vi "Configure.vi"(8 "error in (no error)":errorcluster, 10 "Msg in":T1, 11 "FakePressureController in":refnum<class "TapeMonitor.lvclass">) -> (0 "error out":errorcluster, 1 "new command":string, 2 "Msg out":T1, 3 "FakePressureController out":refnum<class "TapeMonitor.lvclass">)   [LabVIEW 2013, in "TapeMonitor.lvclass"]
uses:
  TapeMonitor.lvclass
  DriverMsg.ctl
  TapeMonitor.lvclass/TapeMonitor.ctl
  OnOffTypeDef.ctl
  source/Device Driver/BaseDriver/BaseDriver.lvclass
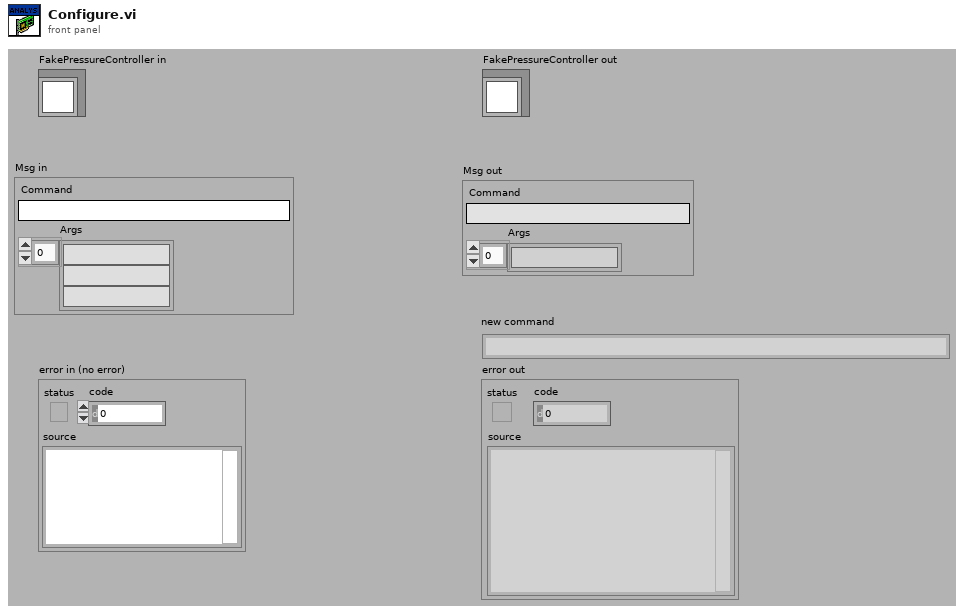
[diagram p1: front panel]
types:
  T1 = typedef "DriverMsg.ctl" = cluster{"Command":string, "Args":string[]}
  T2 = typedef "OnOffTypeDef.ctl" = enum16{"off", "on"}
  T3 = typedef "TapeMonitor.lvclass/settings_TypDef.ctl" = cluster{"timeout":T4, "FitnessLimit":T4, "LocalSavingPath":path, "Save":T2, "threshold_low":T4, "threshold_high":T4, "area_min":T4, "area_max":T4}
  T4 = typedef "BaseDriver.lvclass/numericVariable_TypeDef.ctl" = cluster{"Value":dbl, "Min":dbl, "Max":dbl, "StepSize":dbl, "Tolerance":dbl, "ValueActual":dbl}
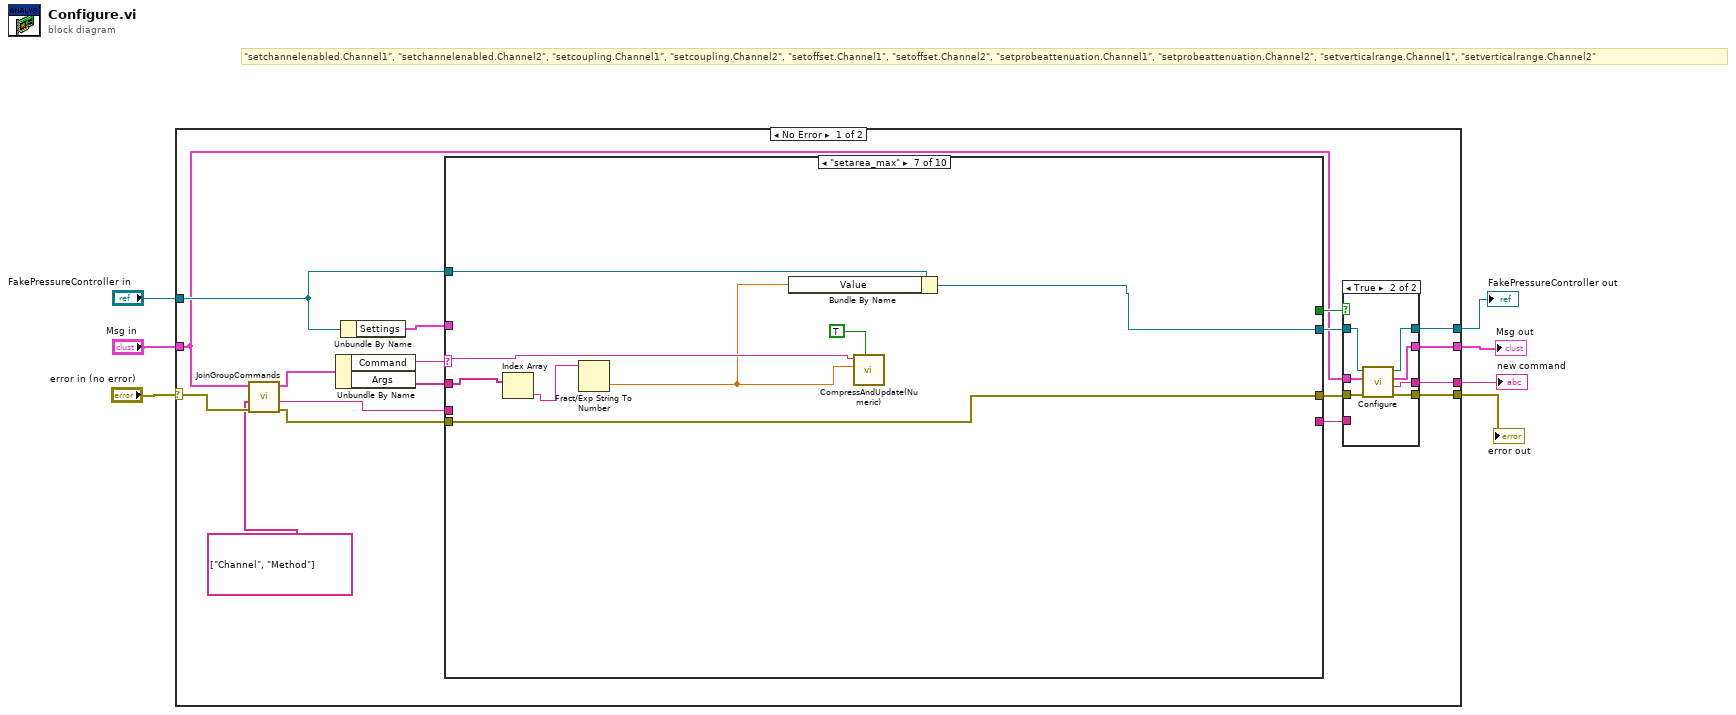
[diagram p0: block diagram]
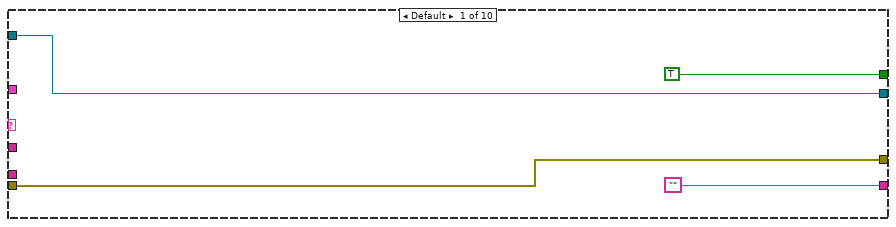
[diagram p3: hidden frame]
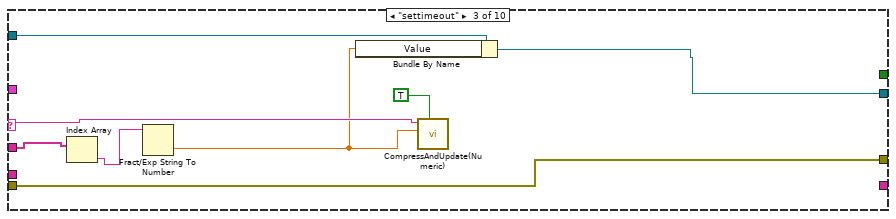
[diagram p5: hidden frame]
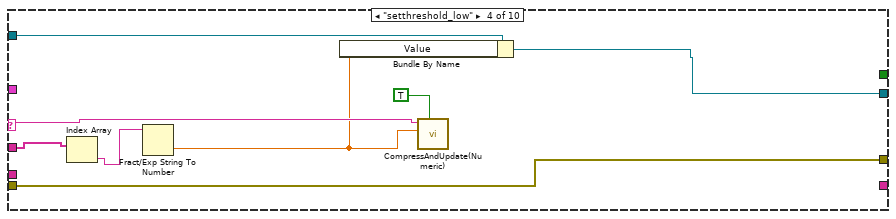
[diagram p6: hidden frame]
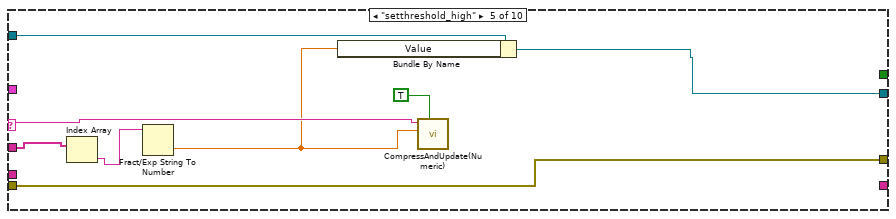
[diagram p7: hidden frame]
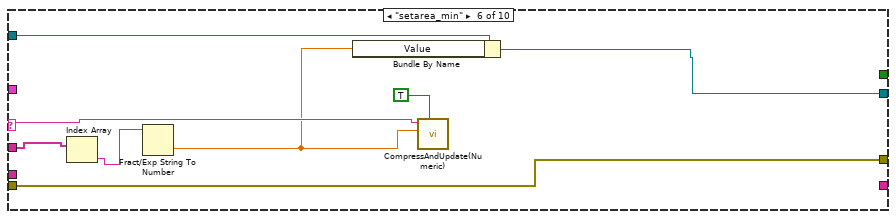
[diagram p8: hidden frame]
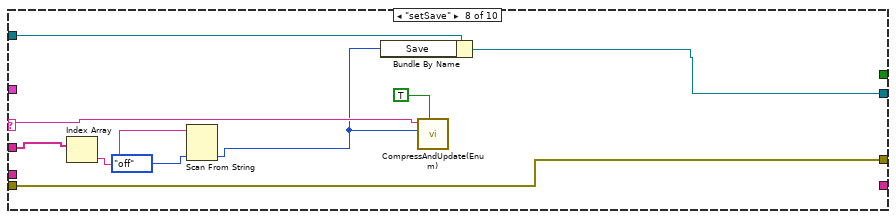
[diagram p9: hidden frame]
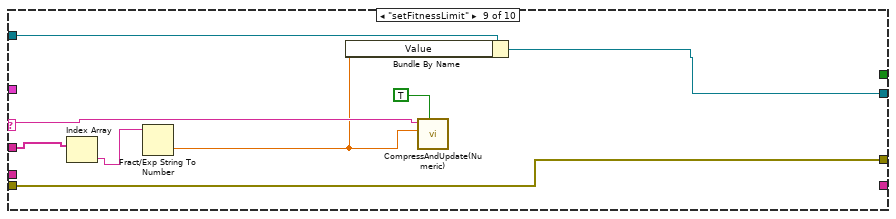
[diagram p10: hidden frame]
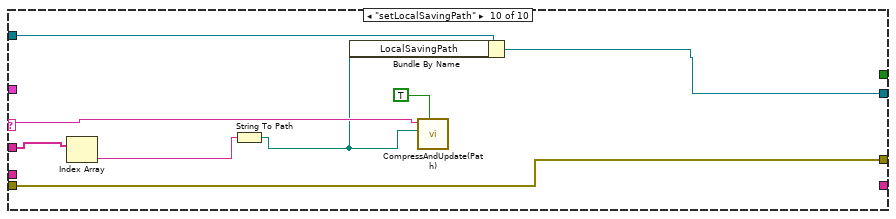
[diagram p11: hidden frame]
diagram:
  # "\"setchannelenabled.Channel1\", \"setchannelenabled.Channel2\", \"setcoupling.Channel1\", \"setcoupling.Channel2\", \"setoffset.Channel1\", \"setoffset.Channel2\", \"setprobeattenuation.Channel1\", \"setprobeattenuation.Channel2\", \"setverticalrange.Channel1\", \"setverticalrange.Channel2\""
  n1 = case shown="No Error" "error in (no error)" {
    selector: "error in (no error)" -> [w13 w110]
    tunnel: "FakePressureController in" -> [w16 w108]
    tunnel: [w24 w108] -> w4
    tunnel: [w22 w110] -> w1
    tunnel: "Msg in" -> [w10 w109]
    tunnel: [w20 w109] -> w3
    tunnel: [w18 _] -> w2
    frame No Error {
      n2 = call "JoinGroupCommands.vi"("error in (no error)"=w13, "Seperator"=string[] ["Channel", "Method"], "Msg in"=w10) -> ("error out"=w12:errorcluster, "Seperator out"=w9:string, "Msg out"=w11:T1)  [unwired: 6 in]
      n3 = Unbundle By Name(w11) -> ("Command"=w17:string, "Args"=w14:string[])
      n4 = Unbundle By Name(w16) -> ("Settings"=w15:T3)
      n5 = case shown="\"setarea_max\"" w17 {
        selector: w17 -> [_ _ w44 w52 w60 w68 w76 w86 w93 w102]
        tunnel: w12 -> [w39 w41 w50 w58 w66 w74 w82 w91 w99 w107]
        tunnel: w14 -> [_ _ w49 w57 w65 w73 w81 w90 w98 w106]
        tunnel: w16 -> [w40 w42 w47 w55 w63 w71 w79 w89 w96 w105]
        tunnel: [w40 w42 w46 w54 w62 w70 w78 w88 w95 w104] -> w25
        tunnel: ["" ("Complete") _ _ _ _ _ _ _ _ _] -> w19
        tunnel: [w39 w41 w50 w58 w66 w74 w82 w91 w99 w107] -> w23
        tunnel: [TRUE _ _ _ _ _ _ _ _ _] -> w21
        tunnel: w15 -> [_ _ _ _ _ _ _ _ _ _]
        tunnel: w9 -> [_ _ _ _ _ _ _ _ _ _]
        frame Default {
        }
        frame "Abort" {
        }
        frame "settimeout" {
          n6 = Index Array(array=w49) -> (element=w48:string)  [unwired: 1 in]
          n7 = Fract/Exp String To Number(string=w48) -> (number=w43:dbl)  [unwired: 3 in, 1 out]
          n8 = Bundle By Name(cluster=w47, "Value"=w43) -> (w46:refnum<class "TapeMonitor.lvclass">)
          n9 = call "CompressAndUpdate(Numeric).vi"("force CVT update (false)"=TRUE, "Numeric"=w43, "command or variable name"=w44) -> ()  [unwired: 8 in, 1 out]
        }
        frame "setthreshold_low" {
          n10 = Index Array(array=w57) -> (element=w56:string)  [unwired: 1 in]
          n11 = Fract/Exp String To Number(string=w56) -> (number=w51:dbl)  [unwired: 3 in, 1 out]
          n12 = Bundle By Name(cluster=w55, "Value"=w51) -> (w54:refnum<class "TapeMonitor.lvclass">)
          n13 = call "CompressAndUpdate(Numeric).vi"("force CVT update (false)"=TRUE, "Numeric"=w51, "command or variable name"=w52) -> ()  [unwired: 8 in, 1 out]
        }
        frame "setthreshold_high" {
          n14 = Index Array(array=w65) -> (element=w64:string)  [unwired: 1 in]
          n15 = Fract/Exp String To Number(string=w64) -> (number=w59:dbl)  [unwired: 3 in, 1 out]
          n16 = Bundle By Name(cluster=w63, "Value"=w59) -> (w62:refnum<class "TapeMonitor.lvclass">)
          n17 = call "CompressAndUpdate(Numeric).vi"("force CVT update (false)"=TRUE, "Numeric"=w59, "command or variable name"=w60) -> ()  [unwired: 8 in, 1 out]
        }
        frame "setarea_min" {
          n18 = Index Array(array=w73) -> (element=w72:string)  [unwired: 1 in]
          n19 = Fract/Exp String To Number(string=w72) -> (number=w67:dbl)  [unwired: 3 in, 1 out]
          n20 = Bundle By Name(cluster=w71, "Value"=w67) -> (w70:refnum<class "TapeMonitor.lvclass">)
          n21 = call "CompressAndUpdate(Numeric).vi"("force CVT update (false)"=TRUE, "Numeric"=w67, "command or variable name"=w68) -> ()  [unwired: 8 in, 1 out]
        }
        frame "setarea_max" {
          n22 = Index Array(array=w81) -> (element=w80:string)  [unwired: 1 in]
          n23 = Fract/Exp String To Number(string=w80) -> (number=w75:dbl)  [unwired: 3 in, 1 out]
          n24 = Bundle By Name(cluster=w79, "Value"=w75) -> (w78:refnum<class "TapeMonitor.lvclass">)
          n25 = call "CompressAndUpdate(Numeric).vi"("force CVT update (false)"=TRUE, "Numeric"=w75, "command or variable name"=w76) -> ()  [unwired: 8 in, 1 out]
        }
        frame "setSave" {
          n26 = Index Array(array=w90) -> (element=w85:string)  [unwired: 1 in]
          n27 = Scan From String(input string=w85, default 1=OnOffTypeDef."off" ("Save")) -> (output 1=w83:T2)  [unwired: 3 in, 3 out]
          n28 = Bundle By Name(cluster=w89, "Save"=w83) -> (w88:refnum<class "TapeMonitor.lvclass">)
          n29 = call "CompressAndUpdate(Enum).vi"("force CVT update (false)"=TRUE, "enum variant"=w83, "command or variable name"=w86) -> ()  [unwired: 8 in, 1 out]
        }
        frame "setFitnessLimit" {
          n30 = Index Array(array=w98) -> (element=w97:string)  [unwired: 1 in]
          n31 = Fract/Exp String To Number(string=w97) -> (number=w92:dbl)  [unwired: 3 in, 1 out]
          n32 = Bundle By Name(cluster=w96, "Value"=w92) -> (w95:refnum<class "TapeMonitor.lvclass">)
          n33 = call "CompressAndUpdate(Numeric).vi"("force CVT update (false)"=TRUE, "Numeric"=w92, "command or variable name"=w93) -> ()  [unwired: 8 in, 1 out]
        }
        frame "setLocalSavingPath" {
          n34 = Index Array(array=w106) -> (element=w100:string)  [unwired: 1 in]
          n35 = String To Path(string=w100) -> (path=w101:path)
          n36 = Bundle By Name(cluster=w105, "LocalSavingPath"=w101) -> (w104:refnum<class "TapeMonitor.lvclass">)
          n37 = call "CompressAndUpdate(Path).vi"("force CVT update (false)"=TRUE, "Path"=w101, "command or variable name"=w102) -> ()  [unwired: 8 in, 1 out]
        }
      }
      n38 = case shown="True" w21 {
        tunnel: w25 -> [w27 w36]
        tunnel: [w27 w35] -> w24
        tunnel: [w28 w34] -> w18
        tunnel: w23 -> [w26 w33]
        tunnel: [w26 w32] -> w22
        tunnel: w10 -> [w29 w31]
        tunnel: [w29 w30] -> w20
        tunnel: w19 -> [w28 _]
        frame False {
        }
        frame True {
          n39 = call-parent "Configure.vi"("error in (no error)"=w33, "Msg in"=w31, "BaseDriver in"=w36) -> ("error out"=w32:errorcluster, "new command"=w34:string, "Msg out"=w30:T1, "BaseDriver out"=w35:refnum<class "TapeMonitor.lvclass">)  [unwired: 5 in]
        }
      }
    }
    frame Error {
    }
  }
  "error out" <- w1
  "FakePressureController out" <- w4
  "new command" <- w2
  "Msg out" <- w3
